vi "Test class line-rate in report.vi"(11 "Test Case In":refnum<class "Coverage Report Test.lvclass">) -> (0 "error out":errorcluster, 3 "Test Case Out":refnum<class "Coverage Report Test.lvclass">)   [LabVIEW 2020, in "Coverage Report Test.lvclass"]
uses:
  Coverage Report Test.lvclass
  Coverage Report Test.lvclass/Coverage Report Test.ctl
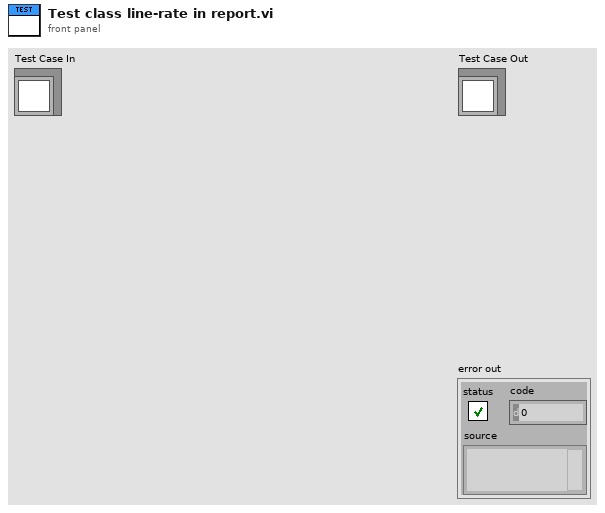
[diagram p1: front panel]
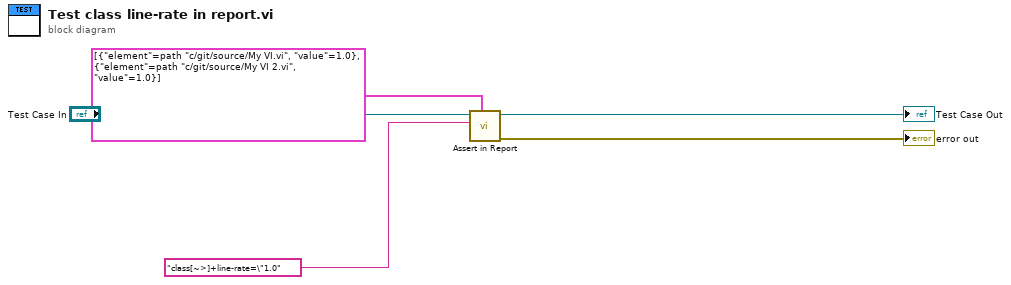
[diagram p0: block diagram]
diagram:
  n1 = call "Assert in Report.vi"("VI:s to Measure"=cluster{"element":path, "value":dbl}[] [{"element"=path "c:/git/source/My VI.vi", "value"=1.0}, {"element"=path "c:/git/source/My VI 2.vi", "value"=1.0}], "Regular Expression"="class[~>]+line-rate=\"1.0", "Coverage Report Test in"="Test Case In") -> ("error out"=→"error out":errorcluster, "Coverage Report Test out"=→"Test Case Out":refnum<class "Coverage Report Test.lvclass">)  [unwired: 7 in]
